vi "06b-arrays.vi"() -> ()   [LabVIEW 2018, in "LV2Julia_examples.lvlib"]
uses:
  LV2Julia_examples.lvlib
  LV2Julia_core/VIs/Server or client state.ctl
  LV2Julia_core/VIs/detailed error info.ctl
  LV2Julia_core/VIs/StackFrame.ctl
  LV2Julia_core/VIs/Commands.ctl
  LV2Julia_core/VIs/ZMQ timeouts.ctl
  0d29fc62-3d1d-4713-a954-9c9e873b3633.vi
  aea790a6-a42b-4eb0-905f-734239196901.vi
  72a46192-383e-4ee5-9465-71670922b82a.vi
  ef5408d4-6538-41d1-b296-fda05a71e4b0.vi
  0fd87d3a-0dd9-45f4-8982-e9f3392e480d.vi
  e4efb182-1b04-4d49-96a3-1defebd055ea.vi
  <vilib>/Analysis/7linalg.llb/Solve Linear Equations (single right hand).vi
  0d29fc62-3d1d-4713-a954-9c9e873b3633.vi/8ee49078-a04b-40cf-aceb-de90d52f19ef.vi
  aea790a6-a42b-4eb0-905f-734239196901.vi/353007a7-a356-474a-8eac-0d4386ef6058.vi
  72a46192-383e-4ee5-9465-71670922b82a.vi/c94a4f76-4d30-4447-b51d-f655efd7ecc9.vi
  ef5408d4-6538-41d1-b296-fda05a71e4b0.vi/1ce3ef63-43bb-49da-8657-644a1439f89e.vi
  0fd87d3a-0dd9-45f4-8982-e9f3392e480d.vi/8f4def8a-33c7-498b-afe1-ab5eba039b80.vi
  e4efb182-1b04-4d49-96a3-1defebd055ea.vi/6dee8664-5f59-405e-8f40-8de208e6b6b2.vi
  e4efb182-1b04-4d49-96a3-1defebd055ea.vi/9d491c07-97c2-4dd2-8657-372a60b757f0.vi
  <vilib>/Analysis/baseanly.llb/Solve Linear Equations By Cholesky.vi
  <vilib>/Analysis/baseanly.llb/Real Matrix to Compact Array.vi
  <vilib>/Analysis/baseanly.llb/Real Compact Tri-Matrix Linear Eqs.vi
  72a46192-383e-4ee5-9465-71670922b82a.vi/c94a4f76-4d30-4447-b51d-f655efd7ecc9.vi/204215fe-ea37-4748-a6af-9cc025445773.vi
  ef5408d4-6538-41d1-b296-fda05a71e4b0.vi/1ce3ef63-43bb-49da-8657-644a1439f89e.vi/4c43ef8e-0dfe-47e4-b073-f55ffa8d1b8c.vi
  0fd87d3a-0dd9-45f4-8982-e9f3392e480d.vi/8f4def8a-33c7-498b-afe1-ab5eba039b80.vi/19d37f1c-5fcd-48b8-9573-300aa88b52d9.vi
  0fd87d3a-0dd9-45f4-8982-e9f3392e480d.vi/8f4def8a-33c7-498b-afe1-ab5eba039b80.vi/e6422bdf-c915-4d44-b9ad-b5de934dbf31.vi
  0fd87d3a-0dd9-45f4-8982-e9f3392e480d.vi/8f4def8a-33c7-498b-afe1-ab5eba039b80.vi/a41177c2-18af-4fd2-8452-b7e4686dcd32.vi
  e4efb182-1b04-4d49-96a3-1defebd055ea.vi/6dee8664-5f59-405e-8f40-8de208e6b6b2.vi/85f272c2-124a-418b-aaf7-baf4275ecbce.vi
  e4efb182-1b04-4d49-96a3-1defebd055ea.vi/6dee8664-5f59-405e-8f40-8de208e6b6b2.vi/c78b0d6d-a63f-49a0-8496-2b24594a6ff7.vi
  72a46192-383e-4ee5-9465-71670922b82a.vi/c94a4f76-4d30-4447-b51d-f655efd7ecc9.vi/204215fe-ea37-4748-a6af-9cc025445773.vi/3e0bbcef-2ee4-4c70-9a45-252a94368a9b.vi
  ef5408d4-6538-41d1-b296-fda05a71e4b0.vi/1ce3ef63-43bb-49da-8657-644a1439f89e.vi/4c43ef8e-0dfe-47e4-b073-f55ffa8d1b8c.vi/9a9e1593-1514-4026-a0eb-3eda3070b93b.vi
  e4efb182-1b04-4d49-96a3-1defebd055ea.vi/6dee8664-5f59-405e-8f40-8de208e6b6b2.vi/85f272c2-124a-418b-aaf7-baf4275ecbce.vi/c96c619f-9d72-4c42-b773-5b49953020e8.vi
  LV2Julia_core/VIs/jl-scripts path.vi
  LV2Julia_core/VIs/check ID validity.vi
  LV2Julia_core/VIs/bindata_descr to JSON.vi
  LV2Julia_core/VIs/check cluster field names.vi
  LV2Julia_core/VIs/concat JSON.vi
  LV2Julia_core/VIs/build request.vi
  LV2Julia_core/VIs/Parse server response.vi
  LV2Julia_core/VIs/log jl exceptions.vi
  <vilib>/Utility/error.llb/Error Cluster From Error Code.vi
  <vilib>/Analysis/7linalg.llb/Solve Linear Eqs (General).vi
  <vilib>/Analysis/7linalg.llb/Solve Linear Eqs (Gen, single right hand).vi
  LV2Julia_core/LV2Julia_core.lvlib
  <vilib>/Analysis/NI_AALPro.lvlib
panel:
  out "LV computation time":dbl
  in  "compare with LV computation":bool=TRUE
  out "Julia roundtrip time (ms)":dbl format="%#.3f"
  out "max difference LV-Jl":dbl format="%#_3e"
  in  "arr size N":u16=4
  out "Solution Vector":dbl[](array[numeric]) format="%.2f"
  out "Known Vector":dbl[](array[numeric])=[22.0, 14.0, 18.0]
  out "Input Matrix (NxN)":dbl[][](array[numeric])=[[1.0, 0.0, 5.0], [4.0, 2.0, 1.0], [2.0, 2.0, 3.0]]
  in  "next":bool
  out "detailed error info":T1
  out "current error":errorcluster
  out "final error":errorcluster
  out "short err code":u8
  in  "stop":bool
  out "ZMQ timeout":bool
  out "Julia script file path":path
  out "temporary script path":path
  out "Jl Server state":T3
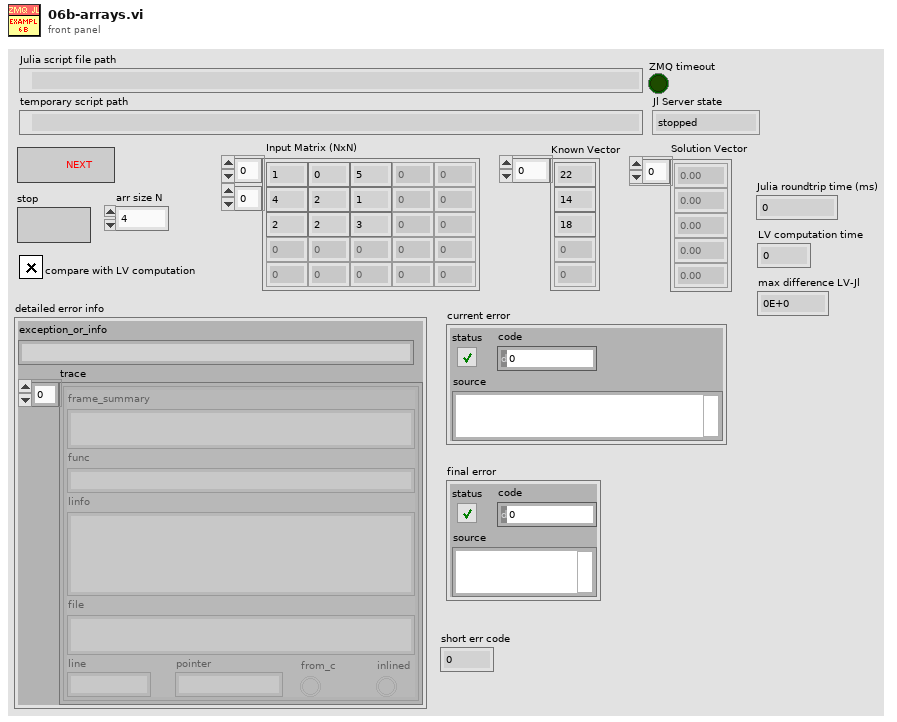
[diagram p1: front panel]
types:
  T1 = typedef "LV2Julia_core.lvlib/detailed error info.ctl" = cluster{"exception_or_info":string, "trace":T2[]}
  T2 = typedef "LV2Julia_core.lvlib/StackFrame.ctl" = cluster{"frame_summary":string, "func":string, "linfo":string, "file":string, "line":i32, "pointer":u64, "from_c":bool, "inlined":bool}
  T3 = typedef "LV2Julia_core.lvlib/Server or client state.ctl" = enum16{"stopped", "running", "unknown"}
  T4 = typedef "LV2Julia_core.lvlib/ZMQ timeouts.ctl" = cluster{"SNDTIMEO":i32, "RCVTIMEO":i32}
  T5 = typedef "LV2Julia_core.lvlib/Commands.ctl" = enum16{"Start Jl-server & Init LV-client", "Send request & Get response ", "Stop Jl-server & Cleanup LV-client", "Cleanup LV-client", "Start Jl-server", "Stop Jl-server", "Init LV-Client", "Cleanup LV-Client", "(not allowed)", "Set LV Client state", "Set Jl Server state", "set ZMQ timeout", "read ZMQ timeout", "read-out state"}
  T6 = typedef "LV2Julia_core.lvlib/Bindata&description.ctl" = cluster{"bindata_descr":T7[], "bindata":u8[]}
  T7 = typedef "LV2Julia_core.lvlib/Bindata description.ctl" = cluster{"nofbytes":i32, "numtype":string, "start":i32, "arrdims":i32[], "kwarg_name":string, "category":string}
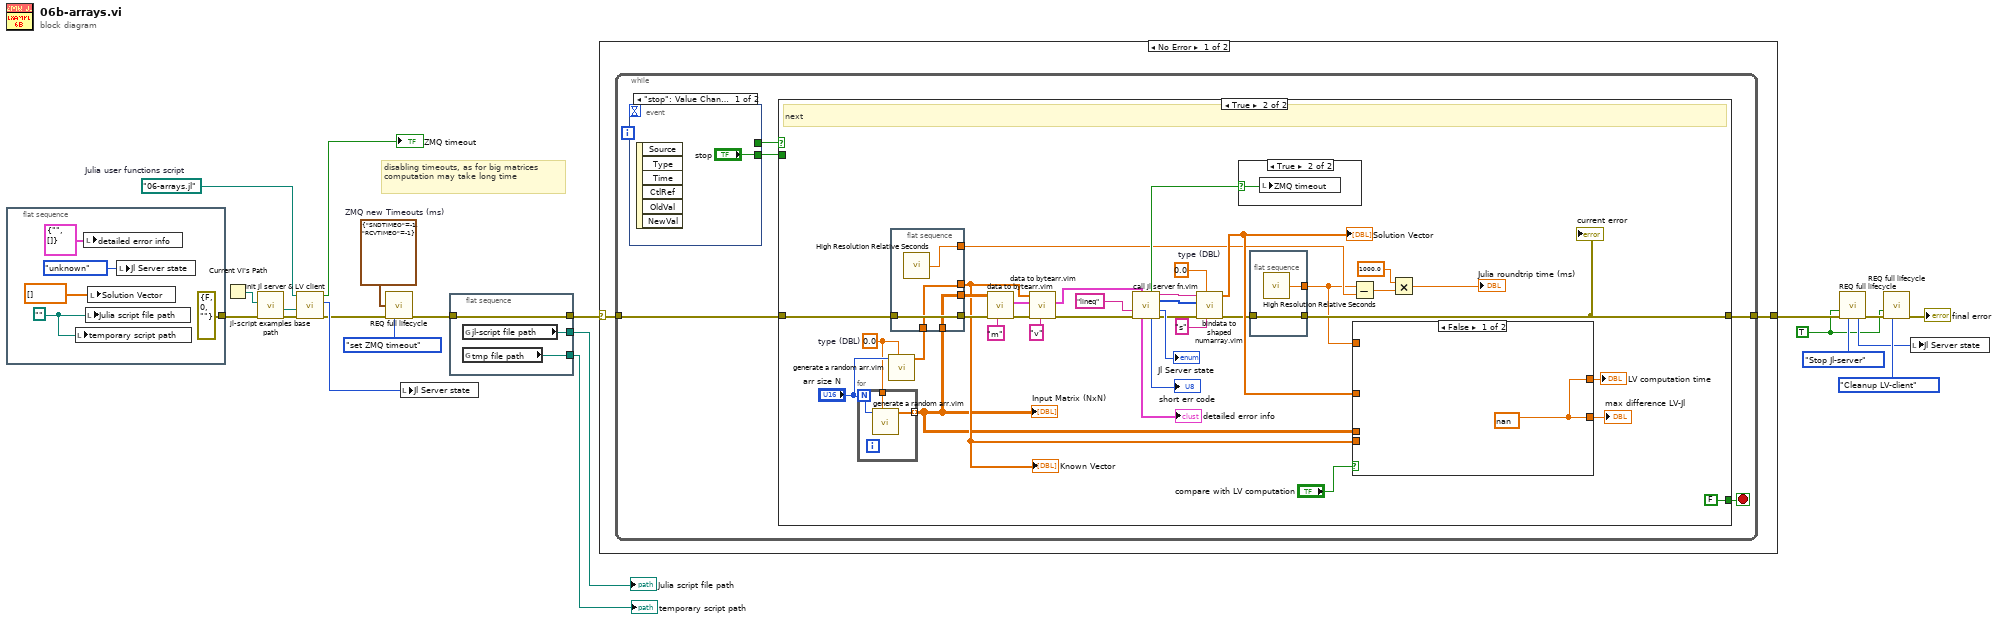
[diagram p0: block diagram]
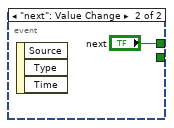
[diagram p2: hidden frame]
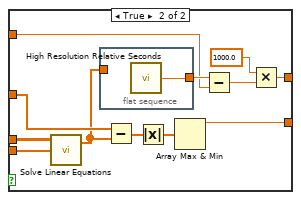
[diagram p4: hidden frame]
diagram:
  w10 = T4 {"SNDTIMEO"=-1, "RCVTIMEO"=-1}  # ZMQ new Timeouts (ms)
  w8 = path "06-arrays.jl"  # Julia user functions script
  w12 = TRUE ("Force command")
  # "disabling timeouts, as for big matrices computation may take long time"
  n1 = flat-sequence {
    tunnel: [errorcluster {"status"=FALSE, "code"=0, "source"=""} ("error in (no error)")] -> w2
    frame #0 {
      w22 = path ""
      n2 = local write "temporary script path"(w22) -> ()
      n3 = local write "detailed error info"(T1 {"exception_or_info"="", "trace"=[]} ("detailed error info")) -> ()
      n4 = local write "Julia script file path"(w22) -> ()
      n5 = local write "Solution Vector"(dbl[] [] ("Server response")) -> ()
      n6 = local write "Jl Server state"(Server_or_client_state."unknown" ("Jl Server state out")) -> ()
    }
  }
  n7 = Current VI's Path() -> (path=w4:path)
  n8 = call "jl-script examples base path.vi"("error in (no error)"=w2, "calling example VI path"=w4) -> ("error out"=w3:errorcluster, "jl-script-examples base path"=w1:path)  [unwired: 8 in]
  n9 = call "init Jl server & LV client.vi"("error in (no error)"=w3, "Base path (not a path)"=w1, "Julia user functions script"=w8) -> ("error out"=w5:errorcluster, "Jl Server state out"=w6:T3, "timeout?"=→"ZMQ timeout":bool)  [unwired: 6 in]
  n10 = call "REQ full lifecycle.vi"("ZMQ new Timeouts in"=w10, "error in"=w5, "command"=Commands."set ZMQ timeout") -> ("error out"=w9:errorcluster)  [unwired: 6 in, 6 out]
  n11 = local write "Jl Server state"(w6) -> ()
  n12 = flat-sequence {
    tunnel: [w29] -> w16
    tunnel: w9 -> [w29]
    tunnel: [w28] -> w14
    tunnel: [w27] -> w15
    frame #0 {
      n13 = global read "jl-scripts path.vi" "jl-script file path"() -> (w28:path)
      n14 = global read "jl-scripts path.vi" "tmp file path"() -> (w27:path)
    }
  }
  n15 = case shown="No Error" w16 {
    selector: w16 -> [w30 w101]
    tunnel: [w31 w101] -> w21
    frame No Error {
      n16 = while {
        tunnel: w30 -> [w35]
        tunnel: [w36] -> w31
        stop <- w33 stop-if-true
        n17 = event shown="[0] \"stop\": Value Change" {
          selector: _ -> [_ _]
          dyn-events: _ -> [_ _]
          timeout: _ -> [_ _]
          tunnel: [_ "next"] -> w34
          tunnel: ["stop" _] -> w32
          event "stop": Value Change {
            n18 = event-data() -> ()  [unwired: 1 in, 6 out]
          }
          event "next": Value Change {
            n19 = event-data() -> ()  [unwired: 1 in, 3 out]
          }
        }
        n20 = case shown="True" w34 {
          tunnel: [w40 w50] -> w36
          tunnel: w35 -> [w40 w55]
          tunnel: [w39 FALSE ("stop this VI only")] -> w33
          tunnel: w32 -> [w39 _]
          frame False {
            # "stop"
          }
          frame True {
            w68 = 0.0  # type (DBL)
            w71 = 0.0  # type (DBL)
            # "next"
            n21 = for {
              N: "arr size N" -> [w97]
              tunnel: [w99] -> w43 mode=indexing
              tunnel: w68 -> [w98]
              n22 = call "generate a random arr.vim"("type in"=w98, "arr size"=w97) -> ("float out"=w99:dbl[])  [unwired: 5 in, 4 out]
            }
            "Input Matrix (NxN)" <- w43
            n23 = call "generate a random arr.vim"("type in"=w68, "arr size"="arr size N") -> ("float out"=w52:dbl[])  [unwired: 5 in, 4 out]
            n24 = flat-sequence {
              tunnel: [w96] -> w54
              tunnel: w55 -> [w96]
              tunnel: w43 -> [w95]
              tunnel: [w95] -> w53
              tunnel: [w94] -> w44
              tunnel: w52 -> [w94]
              tunnel: [w93] -> w49
              frame #0 {
                n25 = call <vilib>:"High Resolution Relative Seconds.vi"() -> ("relative seconds"=w93:dbl)
              }
            }
            n26 = call "data to bytearr.vim"("kwarg_name"="m", "error in (no error)"=w54, "data in"=w53) -> ("error out"=w75:errorcluster, "Bindata & descr out"=w74:T6)  [unwired: 6 in, 1 out]
            n27 = call "data to bytearr.vim"("kwarg_name"="v", "error in (no error)"=w75, "Bindata & descr in"=w74, "data in"=w44) -> ("error out"=w56:errorcluster, "Bindata & descr out"=w60:T6)  [unwired: 5 in, 1 out]
            n28 = call "call Jl server fn.vim"("Bindata & descr in"=w60, "fun2call"="lineq" ("Julia function name"), "error in (no error)"=w56) -> ("timeout?"=w59:bool, "JSON received"=w58:string, "binary data received"=w57:u8[], "Jl Server state out"=→"Jl Server state":T3, "detailed error info"=→"detailed error info":T1, "return code"=→"short err code":u8, "error out"=w61:errorcluster)  [unwired: 6 in]
            n29 = call "bindata to shaped numarray.vim"("name"="s" ("kwarg_name"), "element type"=w71, "error in (no error)"=w61, "binary data"=w57, "JSON in"=w58) -> ("error out"=w51:errorcluster, "numarray 1D"=w67:dbl[])  [unwired: 3 in, 2 out]
            "Solution Vector" <- w67
            n30 = case shown="True" w59 {
              selector: w59 -> [_ w100]
              frame False {
              }
              frame True {
                n31 = local write "ZMQ timeout"(w100) -> ()
              }
            }
            n32 = flat-sequence {
              tunnel: [w92] -> w50
              tunnel: w51 -> [w92]
              tunnel: [w91] -> w42
              frame #0 {
                n33 = call <vilib>:"High Resolution Relative Seconds.vi"() -> ("relative seconds"=w91:dbl)
              }
            }
            n34 = Subtract(x=w42, y=w49) -> (x-y=w47:dbl)
            n35 = case shown="False" "compare with LV computation" {
              tunnel: w67 -> [_ w89]
              tunnel: [w77 w86] -> w66
              tunnel: w43 -> [_ w85]
              tunnel: w44 -> [_ w84]
              tunnel: w42 -> [_ w79]
              tunnel: [w77 w78] -> w41
              frame False {
                w77 = nan
              }
              frame True {
                n36 = call-poly <vilib>:"Solve Linear Equations.vi"("Known Vector"=w84, "Input Matrix"=w85) -> ("Solution Vector"=w83:dbl[])  [unwired: 1 in, 1 out]
                n37 = flat-sequence {
                  tunnel: w83 -> [_]
                  tunnel: [w90] -> w80
                  frame #0 {
                    n38 = call <vilib>:"High Resolution Relative Seconds.vi"() -> ("relative seconds"=w90:dbl)
                  }
                }
                n39 = Subtract(x=w89, y=w83) -> (x-y=w88:dbl[])
                n40 = Absolute Value(x=w88) -> (abs(x)=w87:dbl[])
                n41 = Array Max & Min(array=w87) -> (max value=w86:dbl)  [unwired: 3 out]
                n42 = Subtract(x=w80, y=w79) -> (x-y=w81:dbl)
                n43 = Multiply(x=1000.0, y=w81) -> (x*y=w78:dbl)
              }
            }
            "max difference LV-Jl" <- w66
            "LV computation time" <- w41
            n44 = Multiply(x=1000.0, y=w47) -> (x*y=→"Julia roundtrip time (ms)":dbl)
            "current error" <- w50
            "Known Vector" <- w44
          }
        }
      }
    }
    frame Error {
    }
  }
  n45 = call "REQ full lifecycle.vi"("Force command"=w12, "error in"=w21, "command"=Commands."Stop Jl-server") -> ("Jl Server state out"=w13:T3, "error out"=w19:errorcluster)  [unwired: 6 in, 5 out]
  n46 = call "REQ full lifecycle.vi"("Force command"=w12, "error in"=w19, "command"=Commands."Cleanup LV-client") -> ("error out"=→"final error":errorcluster)  [unwired: 6 in, 6 out]
  n47 = local write "Jl Server state"(w13) -> ()
  "temporary script path" <- w15
  "Julia script file path" <- w14
